vi "video.property_key_at.vi"(8 "error in":errorcluster, 11 "Video in":refnum<class "Video.lvclass">) -> (0 "error out":errorcluster, 3 "Video out":refnum<class "Video.lvclass">)   [LabVIEW 2020, in "Video.lvclass"]
doc: "Returns the key of the property at the given index."
uses:
  Video.lvclass
  Video.lvclass/Video.ctl
  client.lvlib
panel:
  out "out_needed out":u32
  out "property key":string
  in  "index":i32
  in  "buf":string
  in  "cap":u32
  in  "out_needed":u32
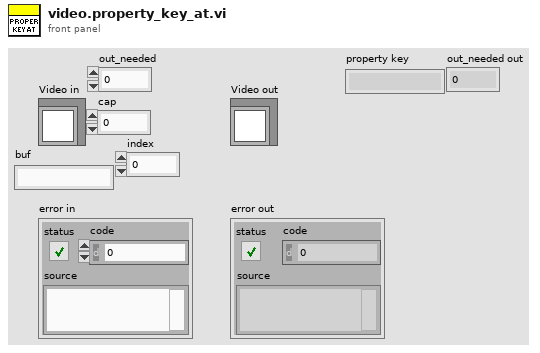
[diagram p1: front panel]
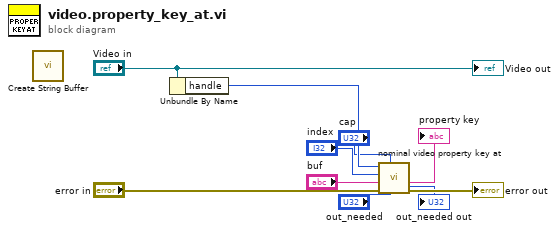
[diagram p0: block diagram]
diagram:
  n1 = call "Create String Buffer.vi"() -> ()  [unwired: 9 in, 3 out]
  n2 = Unbundle By Name("Video in") -> ("handle"=w8:i32)
  n3 = call "nominal video property key at.vi"("out_needed"="out_needed", "cap"="cap", "error in (no error)"="error in", "buf"="buf", "index"="index", "video"=w8) -> ("error out"=→"error out":errorcluster, "buf out"=→"property key":string, "out_needed out"=→"out_needed out":u32)  [unwired: 2 in, 1 out]
  "Video out" <- "Video in"
